vi "Part 1.vi"(11 "Input":string) -> (3 "Output":i64)   [LabVIEW 2021]
uses:
  <userlib>/_OpenG.lib/string/string.llb/Convert EOLs (String)__ogtk.vi
panel:
  out "Array":bool[][](array[boolean])
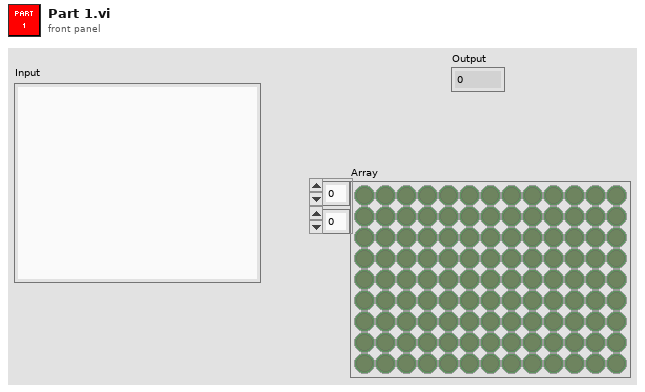
[diagram p1: front panel]
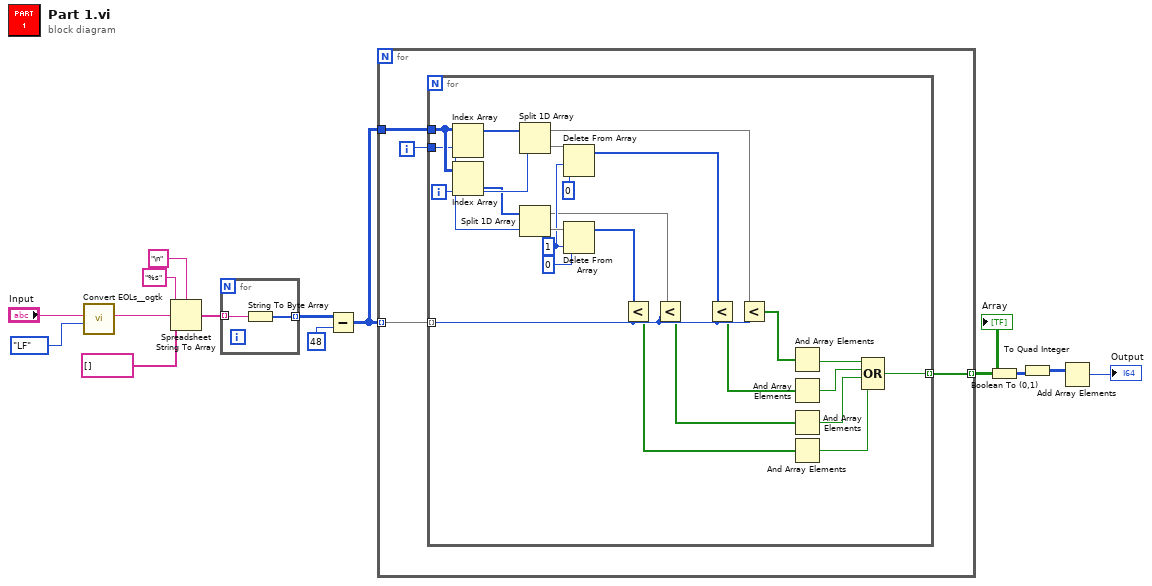
[diagram p0: block diagram]
diagram:
  n1 = call-poly <userlib>:"Convert EOLs__ogtk.vi"("Convert to:"=enum16{"CR", "LF", "CRLF"}."LF", "String in"="Input") -> ("String out"=w10:string)  [unwired: 9 in]
  n2 = Spreadsheet String To Array(delimiter (Tab)="\n", format string="%s", spreadsheet string=w10, array type (2D Dbl)=string[] []) -> (array=w8:string[])
  n3 = for {
    tunnel: w8 -> [w16] mode=indexing
    tunnel: [w15] -> w7 mode=indexing
    n4 = String To Byte Array(string=w16) -> (unsigned byte array=w15:u8[])
  }
  n5 = Subtract(x=w7, y=u8 48) -> (x-y=w5:u8[][])
  n6 = for {
    tunnel: w5 -> [w20] mode=indexing
    tunnel: w5 -> [w19]
    tunnel: [w17] -> w4 mode=indexing
    i -> [w18]
    n7 = for {
      tunnel: w20 -> [w33] mode=indexing
      tunnel: w19 -> [w44]
      tunnel: w18 -> [w40]
      tunnel: [w23] -> w17 mode=indexing
      i -> [w42]
      w37 = 1 ("length")
      n8 = Index Array(array=w44, index (row)=w40) -> (element=w43:u8[])  [unwired: 1 in]
      n9 = Index Array(array=w44, index (col)=w42) -> (element=w41:u8[])  [unwired: 1 in]
      n10 = Split 1D Array(array=w43, index=w42) -> (first subarray=w32:u8[], second subarray=w39:u8[])
      n11 = Split 1D Array(array=w41, index=w40) -> (first subarray=w34:u8[], second subarray=w38:u8[])
      n12 = Delete From Array(array=w39, length=w37, index=0) -> (array with subset deleted=w35:u8[])  [unwired: 1 out]
      n13 = Delete From Array(array=w38, length=w37, index=0) -> (array with subset deleted=w36:u8[])  [unwired: 1 out]
      n14 = Less?(x=w36, y=w33) -> (x < y?=w28:bool[])
      n15 = Less?(x=w34, y=w33) -> (x < y?=w29:bool[])
      n16 = Less?(x=w35, y=w33) -> (x < y?=w30:bool[])
      n17 = Less?(x=w32, y=w33) -> (x < y?=w31:bool[])
      n18 = And Array Elements(Boolean array=w31) -> (logical AND=w24:bool)
      n19 = And Array Elements(Boolean array=w30) -> (logical AND=w25:bool)
      n20 = And Array Elements(Boolean array=w29) -> (logical AND=w26:bool)
      n21 = And Array Elements(Boolean array=w28) -> (logical AND=w27:bool)
      n22 = Compound Arithmetic op=OR(w24, w25, w26, w27) -> (w23:bool)
    }
  }
  "Array" <- w4
  n23 = Boolean To (0,1)(Boolean=w4) -> (0, 1=w3:i16[][])
  n24 = To Quad Integer(1:w3) -> (0:w2:i64[][])
  n25 = Add Array Elements(numeric array=w2) -> (sum=→"Output":i64)
